vi "Get Session Property (DBL).vi"(0 "session in":refnum<k21>, 7 "property":refnum<k21>, 11 "error in (no error)":errorcluster) -> (4 "session out":refnum<k21>, 10 "property value":dbl, 15 "error out":errorcluster)   [LabVIEW 2020, in "SLSC.lvlib"]
uses:
  <vilib>/SLSC/SLSC.lvlib
  nislsclvapi.dll
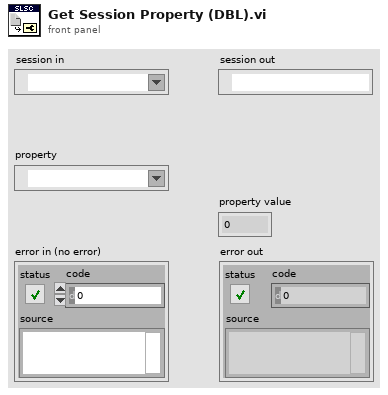
[diagram p1: front panel]
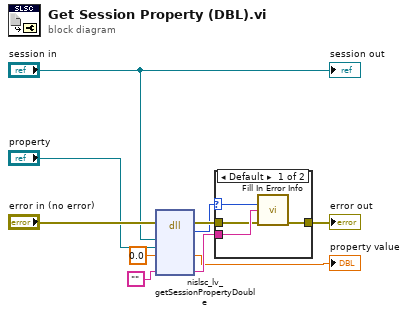
[diagram p0: block diagram]
diagram:
  n1 = dll-call lib="nislsclvapi.*" fn="nislsc_lv_getSessionPropertyDouble"(error in="error in (no error)", "session"="session in", "property"="property", "propertyValue"=0.0, "extendedErrorInfo"="") -> (error out=w7:errorcluster, w6:i32, "propertyValue"=→"property value":dbl, "extendedErrorInfo"=w8:string)  [unwired: 6 in, 1 out]
  n2 = case shown="Default" w6 {
    selector: w6 -> [w14 _]
    tunnel: w8 -> [w13 _]
    tunnel: w7 -> [w12 w15]
    tunnel: [w11 w15] -> w5
    frame Default {
      n3 = call <vilib>:"Fill In Error Info.vi"("status code"=w14, "extended error info"=w13, "error in"=w12) -> ("error out"=w11:errorcluster)  [unwired: 12 in]
    }
    frame 0 {
    }
  }
  "error out" <- w5
  "session out" <- "session in"
